vi "Icon_Write body text.vi"(5 "Color Set":T7, 6 "Frame":T1, 7 "Text Array":T8, 8 "Error":errorcluster, 9 "Region":T2={"Left"=0, "Top"=2, "Right"=0, "Bottom"=0, "Width"=0, "Height"=0, "Start"={"Left"=0, "Top"=0}}, 10 "Line Count":u32, 11 "Icon":T4) -> (0 "Error Out":errorcluster, 2 "Result Array Out":T5[](array[typedef]), 3 "Icon Out":T4 caption="Icon")   [LabVIEW 2014]
uses:
  Controls/Array/String Array_Body Text.ctl
  Controls/String_Picture/STRING_Line Display.ctl
  Controls/Cluster/Cluster_Text Color Set.ctl
  Controls/Cluster/CLuster_Line Fit Results.ctl
  Controls/Enum/ENUM RB_Fit Result.ctl
  Controls/String_Picture/Picture_Icon.ctl
  Controls/Cluster/Cluster_Region info.ctl
  Controls/Cluster/Cluster_Top Left position.ctl
  Controls/Enum/ENUM_Frame Template Select.ctl
  Controls/Enum/ENUM_Text Justify.ctl
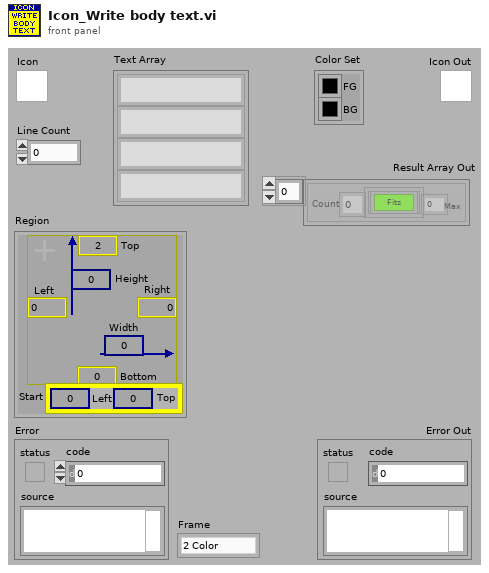
[diagram p1: front panel]
types:
  T1 = typedef "ENUM_Frame Template Select.ctl" = enum16{"2 Color", "5 Color"}
  T2 = typedef "Cluster_Region info.ctl" = cluster{"Left":i32, "Top":i32, "Right":i32, "Bottom":i32, "Width":u32, "Height":u32, "Start":T3}
  T3 = typedef "Cluster_Top Left position.ctl" = cluster{"Left":i32, "Top":i32}
  T4 = typedef "Picture_Icon.ctl" = picture
  T5 = typedef "CLuster_Line Fit Results.ctl" = cluster{"Fit Result":T6, "Max":i32, "Count":i32}
  T6 = typedef "ENUM RB_Fit Result.ctl" = enum32{"Fits", "Almost Fits", "NO Fit"}
  T7 = typedef "Cluster_Text Color Set.ctl" = cluster{"BG":u32, "FG":u32}
  T8 = typedef "String Array_Body Text.ctl" = T9[]
  T9 = typedef "STRING_Line Display.ctl" = string
  T10 = typedef "ENUM_Text Justify.ctl" = enum16{"Left", "Center", "Right"}
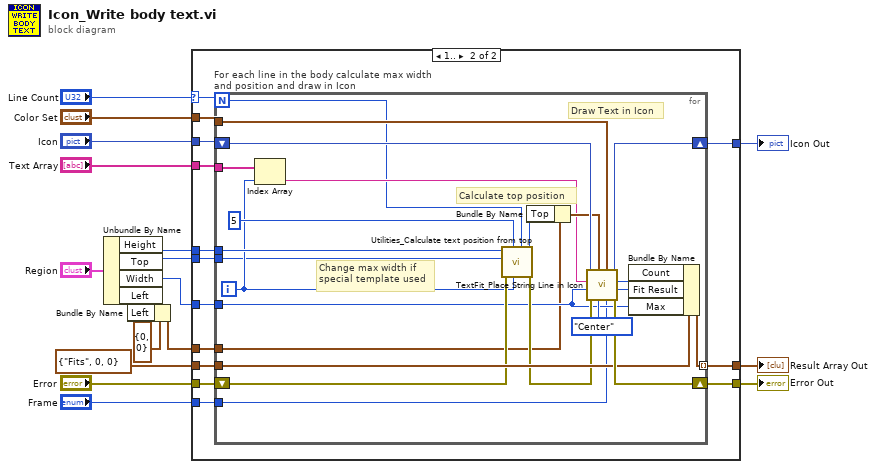
[diagram p0: block diagram]
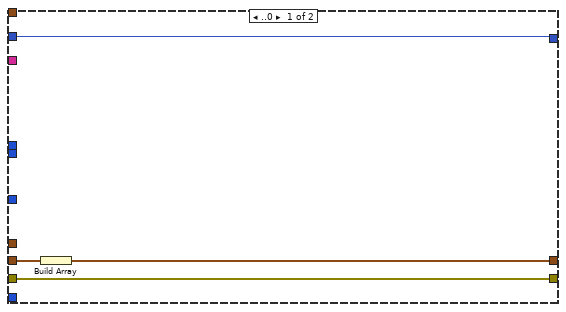
[diagram p2: hidden frame]
diagram:
  n1 = Unbundle By Name("Region") -> ("Height"=w2:u32, "Top"=w6:i32, "Width"=w7:u32, "Left"=w3:i32)
  n2 = Bundle By Name(cluster=T3 {"Left"=0, "Top"=0} ("Starting Positn In"), "Left"=w3) -> (w4:T3)
  n3 = case shown="1.." "Line Count" {
    selector: "Line Count" -> [_ w24]
    tunnel: [w20 w35] -> w9
    tunnel: "Icon" -> [w21 w34]
    tunnel: [w21 w33] -> w11
    tunnel: T5 {"Fit Result"=enum."Fits", "Max"=0, "Count"=0} ("Cluster") -> [w18 w32]
    tunnel: [w19 w31] -> w13
    tunnel: "Color Set" -> [_ w30]
    tunnel: "Error" -> [w20 w29]
    tunnel: w2 -> [_ w28]
    tunnel: w4 -> [_ w27]
    tunnel: w7 -> [_ w26]
    tunnel: "Text Array" -> [_ w25]
    tunnel: w6 -> [_ w23]
    tunnel: "Frame" -> [_ w22]
    frame ..0 {
      n4 = Build Array(w18) -> (w19:T5[])
    }
    frame 1.. {
      n5 = for "For each line in the body calculate max width and position and draw in Icon" {
        N: w24 -> [w39]
        shift-right: [w55] -> w35
        shift-left: w29 -> [w45]
        tunnel: w25 -> [w50]
        shift-right: [w56] -> w33
        shift-left: w34 -> [w57]
        tunnel: w26 -> [w43]
        tunnel: w28 -> [w51]
        tunnel: w27 -> [w38]
        tunnel: w32 -> [w49]
        tunnel: [w48] -> w31 mode=indexing
        tunnel: w30 -> [w42]
        tunnel: w23 -> [w37]
        tunnel: w22 -> [w36]
        i -> [w40]
        # "Draw Text in Icon"
        # "Calculate top position"
        # "Change max width if \nspecial template used"
        n6 = Index Array(array=w50, index=w40) -> (element=w41:T9)
        n7 = call "Utilities_Calculate text position from top.vi"("Line Count"=w39, "Line Index"=w40, "Line Height"=5 ("Line Height In"), "Error"=w45, "Starting Offset"=w37, "Field Total Height"=w51) -> ("Error Out"=w44:errorcluster, "Text Positn From Top Out"=w52:i32)  [unwired: 4 in]
        n8 = Bundle By Name(cluster=w38, "Top"=w52) -> (w53:T3)
        n9 = call "TextFit_Place String Line in Icon.vi"("Frame"=w36, "Color Set"=w42, "Justify"=ENUM_Text_Justify."Center" ("Justify In"), "Starting Position"=w53, "Error"=w44, "Max Width"=w43, "String"=w41, "ICON"=w57) -> ("Error Out"=w55:errorcluster, "Fit Result Out"=w47:T6, "Final Size Out"=w46:i32, "ICON Out"=w56:T4)
        n10 = Bundle By Name(cluster=w49, "Count"=w46, "Fit Result"=w47, "Max"=w43) -> (w48:T5)
      }
    }
  }
  "Result Array Out" <- w13
  "Icon Out" <- w11
  "Error Out" <- w9
